vi "LWXPS_InitializeAndHomeX.vi"(6 "LabVIEW error IN":errorcluster, 8 "Option":string, 9 "XPS Reference IN":refnum<k24>) -> (0 "LabVIEW error OUT":errorcluster, 1 "XPS Error String":string, 2 "Returned error code":i32, 3 "XPS Reference OUT":refnum<k24>)   [LabVIEW 2015]
uses:
  C:/Users/Becky/Desktop/XPS-UNIFIED/LabVIEW VIs/LabVIEW Source Code/Dll/Newport.XPS.CommandInterface.dll
  Dll/Newport.XPS.CommandInterface.dll
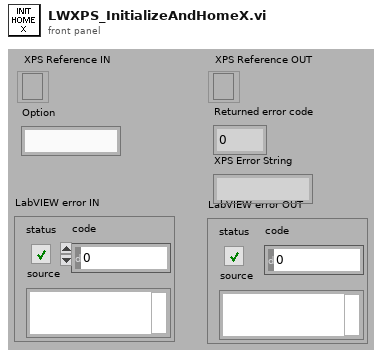
[diagram p1: front panel]
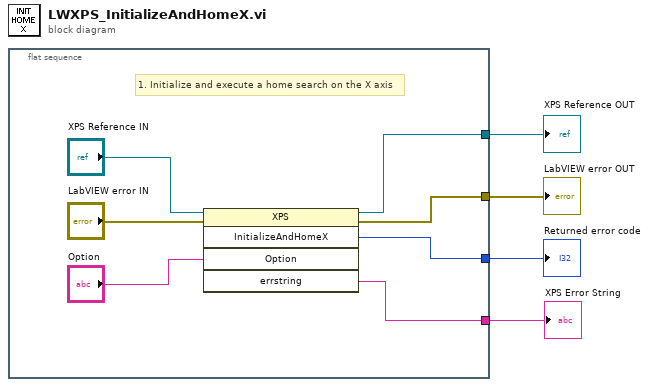
[diagram p0: block diagram]
diagram:
  n1 = flat-sequence {
    tunnel: [w8] -> w4
    tunnel: [w10] -> w3
    tunnel: [w5] -> w2
    tunnel: [w7] -> w1
    frame #0 {
      # "1. Initialize and execute a home search on the X axis"
      n2 = invoke class="XPS" method="InitializeAndHomeX"(reference="XPS Reference IN", error in="LabVIEW error IN", "Option"="Option") -> (reference out=w8:refnum<k24>, error out=w10:errorcluster, "InitializeAndHomeX"=w5:i32, "errstring"=w7:string)  [unwired: 2 in, 1 out]
    }
  }
  "XPS Reference OUT" <- w4
  "LabVIEW error OUT" <- w3
  "Returned error code" <- w2
  "XPS Error String" <- w1
